vi "1-Wire-Read.vi"() -> ()   [LabVIEW 2020]
panel:
  out "Error String":string
  out "error out":errorcluster
  out "aData":u32[](array[numeric]) format="%x"
  out "aValuesOut":u32[](array[numeric]) format="%x"
  in  "Identifier":string="LJM_idANY"
  in  "ConnectionType":string="LJM_ctANY"
  in  "DeviceType":string="LJM_dtANY"
  in  "1-Wire":T1={"SENS"=8, "DPU"=0, "Options"=0, "Function"=85, "Num Tx"=1, "Num Rx"=9, "TX Data"=[190], "ROM H"=838862850, "ROM L"=2946959376, "Branches H"=0, "Branches L"=0, "Search Res H"=0, "Search Res L"=0, "Path H"=0, "Path L"=0} {"Path L" format="%x"; "Path H" format="%x"; "Search Res L" format="%x"; "Search Res H" format="%x"; "Branches L" format="%x"; "Branches H" format="%x"; "ROM L" format="%x"; "ROM H" format="%x"; "TX Data" format="%x"; "Function" format="%x"}
  # "Functions: \nSearch 0xF0\nSkip 0xCC\nMatch 0x55\nRead 0x33"
  # "Searching for a 1-Wire Probe ROM Id:\n1. Configure SENS channel,\n    0: FIO0\n    1: FIO1\n    8: EIO0\n    9: EIO1\n    10: EIO2\n    11: EIO3\n    12: EIO4\n    13: EIO5\n    14: EIO6\n    15: EIO7\n     etc.\n2. Set the \"Functions\" option to 0xF0\n3. Run the .vi\n4. \"ROM H\" reports the upper bytes and \n    \"ROM L\" reports the lower bytes of the \n    1-wire chip ID."
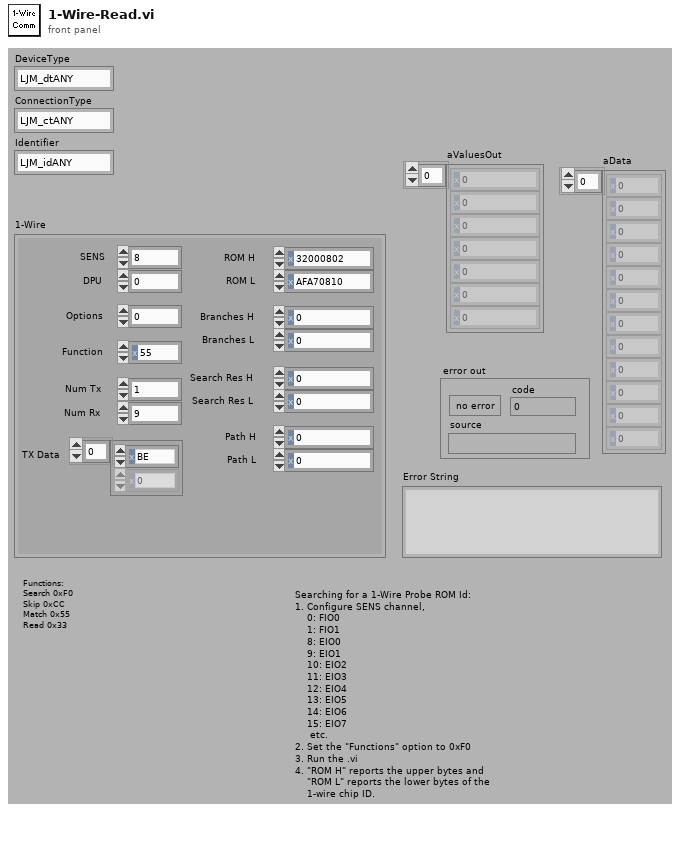
[diagram p1: front panel]
types:
  T1 = cluster{"SENS":u32, "DPU":u32, "Options":u32, "Function":u32, "Num Tx":u32, "Num Rx":u32, "TX Data":u16[], "ROM H":u32, "ROM L":u32, "Branches H":u32, "Branches L":u32, "Search Res H":u32, "Search Res L":u32, "Path H":u32, "Path L":u32}
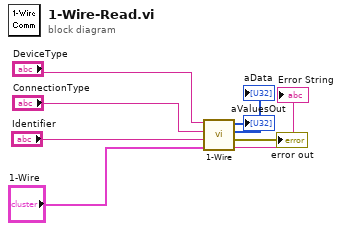
[diagram p0: block diagram]
diagram:
  n1 = call "1-Wire.vi"("1-Wire"="1-Wire", "Identifier"="Identifier", "ConnectionType"="ConnectionType", "DeviceType"="DeviceType") -> ("Error String"=→"Error String":string, "error out"=→"error out":errorcluster, "aData"=→"aData":u32[], "aValuesOut"=→"aValuesOut":u32[])
